vi "Update Measurement UI.vi"(8 "error in (no error)":errorcluster, 11 "Measurement in":refnum<class "Measurement.lvclass">) -> (0 "error out":errorcluster, 3 "Measurement out":refnum<class "Measurement.lvclass">)   [LabVIEW 2017, in "Measurement Actor.lvlib" / "Measurement.lvclass"]
uses:
  Measurement.lvclass
  Measurement.lvclass/Measurement.ctl
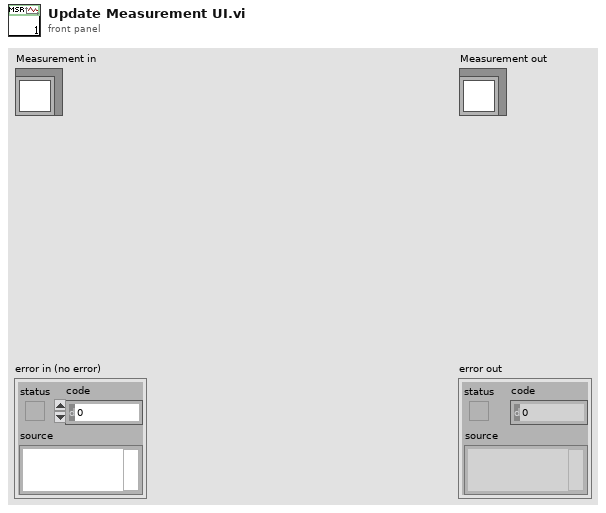
[diagram p1: front panel]
types:
  T1 = typedef "Measurement Actor.lvlib/Measurement.lvclass/Iteration count.ctl" = cluster{"Desired Iterations":i32, "Current":i32}
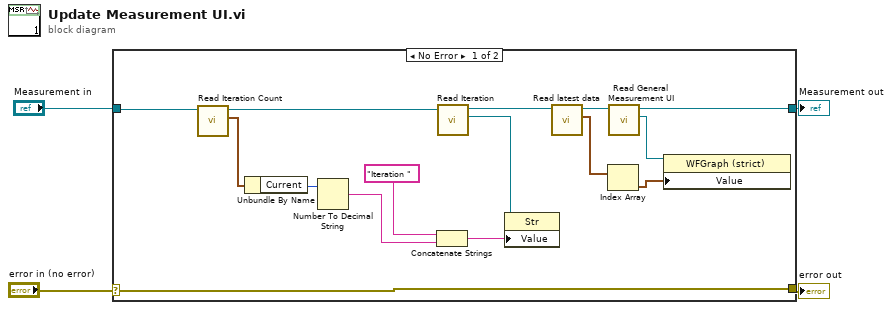
[diagram p0: block diagram]
diagram:
  n1 = case shown="No Error" "error in (no error)" {
    selector: "error in (no error)" -> [w19 w21]
    tunnel: [w19 w21] -> w3
    tunnel: [w8 w20] -> w1
    tunnel: "Measurement in" -> [w10 w20]
    frame No Error {
      n2 = call "Read Iteration Count.vi"("Measurement in"=w10) -> ("Iteration Count"=w18:T1, "Measurement out"=w12:refnum<class "Measurement.lvclass">)  [unwired: 8 in, 1 out]
      n3 = Unbundle By Name(w18) -> ("Current"=w17:i32)
      n4 = Number To Decimal String(number=w17) -> (decimal integer string=w15:string)  [unwired: 1 in]
      n5 = Concatenate Strings("Iteration " ("string"), w15) -> (w14:string)
      n6 = call "Read Iteration.vi"("Measurement in"=w12) -> ("Iteration"=w16:refnum<vi>, "Measurement out"=w11:refnum<class "Measurement.lvclass">)  [unwired: 8 in, 1 out]
      n7 = property class="Str"(reference=w16, "Value"=w14) -> ()  [unwired: 1 in, 2 out]
      n8 = call "Read latest data.vi"("Measurement in"=w11) -> ("latest data"=w6:waveform(dbl)[], "Measurement out"=w9:refnum<class "Measurement.lvclass">)  [unwired: 8 in, 1 out]
      n9 = Index Array(array=w6) -> (element=w5:waveform(dbl))  [unwired: 1 in]
      n10 = call "Read General Measurement UI.vi"("Measurement in"=w9) -> ("General Measurement UI"=w7:refnum<vi>, "Measurement out"=w8:refnum<class "Measurement.lvclass">)  [unwired: 8 in, 1 out]
      n11 = property class="WFGraph (strict)"(reference=w7, "Value"=w5) -> ()  [unwired: 1 in, 2 out]
    }
    frame Error {
    }
  }
  "error out" <- w3
  "Measurement out" <- w1
